vi "TestExample.vi"() -> ()   [LabVIEW 2012, in "Surelite I.lvlib"]
doc: "This is the instrument driver for the <INSTRUMENT NAME>. The VI Tree displays all the user-callable VIs of the instrument driver in an organized table."
uses:
  Surelite I.lvlib
panel:
  in  "ClearErr":bool
  out "error out":errorcluster
  out "Error Message":string[](array[string])
  in  "Check Error":bool
  in  "Shutdown":bool
  in  "Reset":bool
  in  "VISA resource name":refnum<visa-resource-name>="COM8"
  in  "Delay (us)":i32=200
  in  "RepRate (Hz)":sgl=10.0 min=0.1 max=30 step=0.1
  in  "Division":i32=1 min=1
  in  "Start? (F)":bool
  in  "Shutter (F)":bool
  in  "Voltage (kV)":sgl=1.08 min=0.9 max=1.2 step=0.01
  in  "Serial Configuration":T1={"Baud Rate"=9600, "Parity"=0, "Data Bits"=8, "Stop Bits"=10, "Flow Control"=0} {"Flow Control" items=["None", "XON/XOFF", "RTS/CTS", "XON/XOFF & RTS/CTS", "DTR/DSR", "XON/XOFF & DTR/DSR"]; "Stop Bits" items=["1.0"=10, "1.5"=15, "2.0"=20]; "Data Bits" items=["7"=7, "8"=8]; "Parity" items=["None", "Odd", "Even", "Mark", "Space"]; "Baud Rate" items=["300"=300, "600"=600, "1200"=1200, "2400"=2400, "4800"=4800, "9600"=9600, "19200"=19200]}
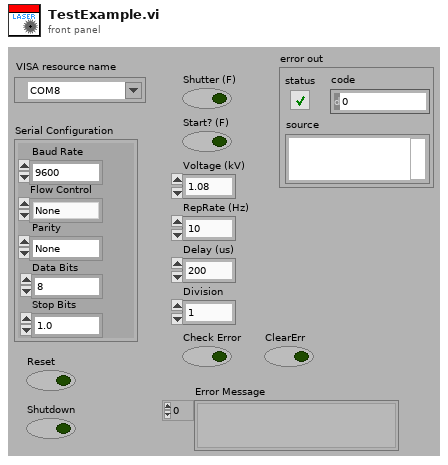
[diagram p1: front panel]
types:
  T1 = cluster{"Baud Rate":u32, "Parity":u16, "Data Bits":u16, "Stop Bits":u16, "Flow Control":u16}
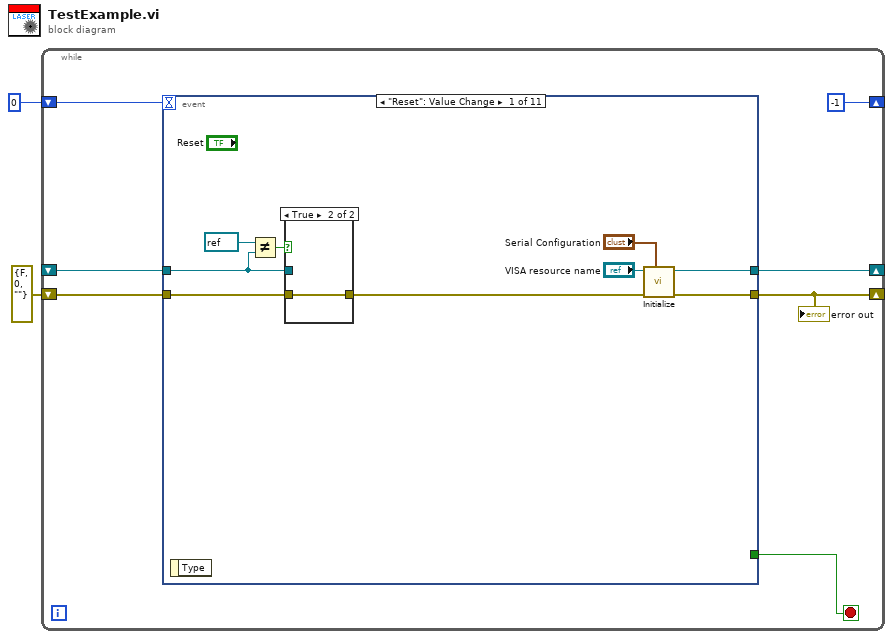
[diagram p0: block diagram]
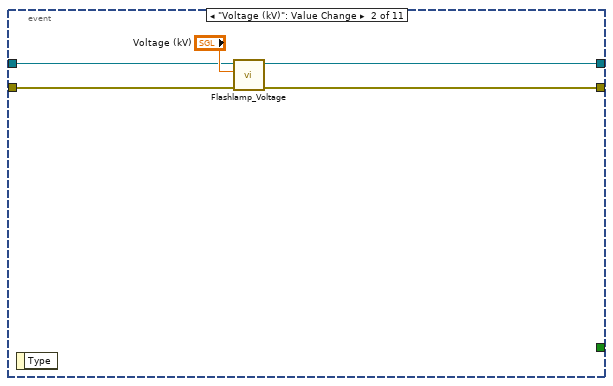
[diagram p3: hidden frame]
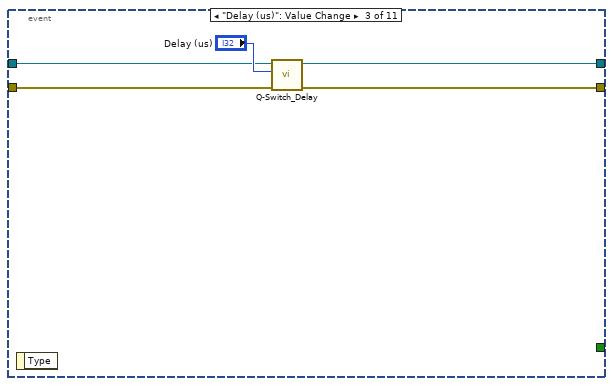
[diagram p4: hidden frame]
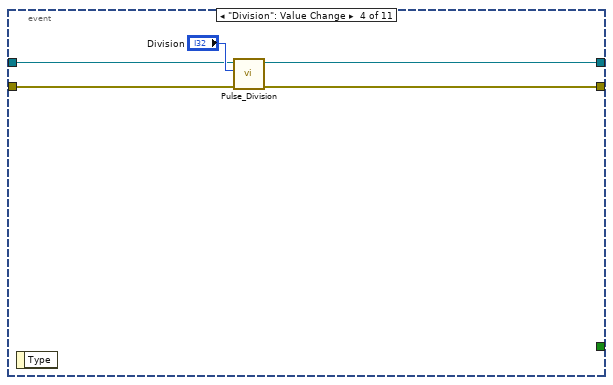
[diagram p5: hidden frame]
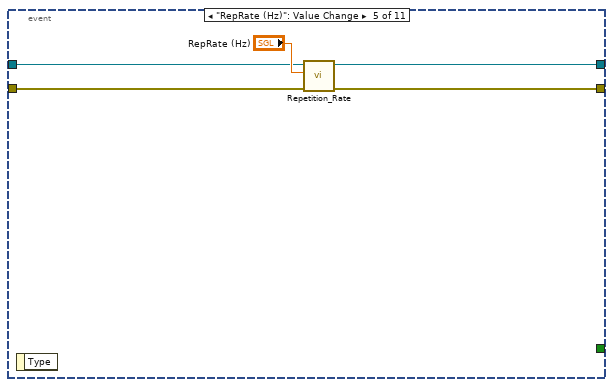
[diagram p6: hidden frame]
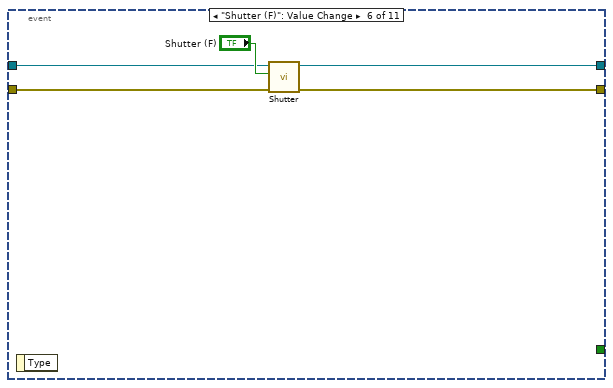
[diagram p7: hidden frame]
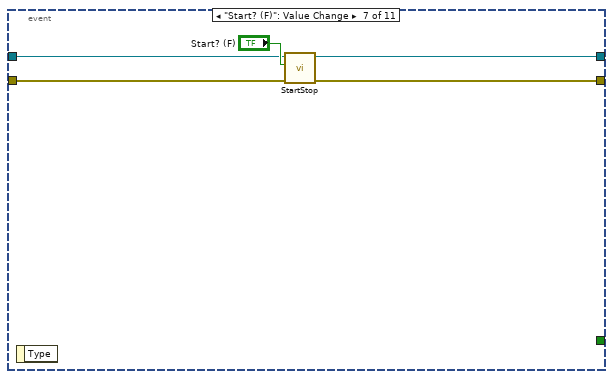
[diagram p8: hidden frame]
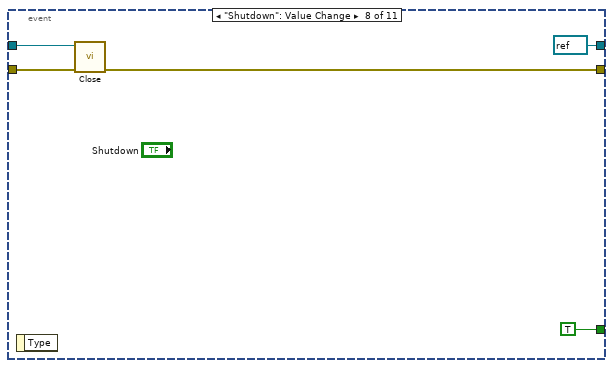
[diagram p9: hidden frame]
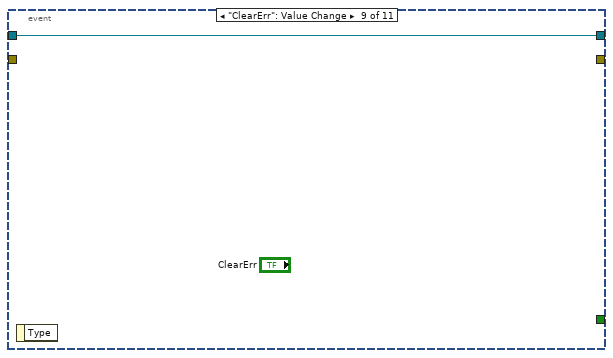
[diagram p10: hidden frame]
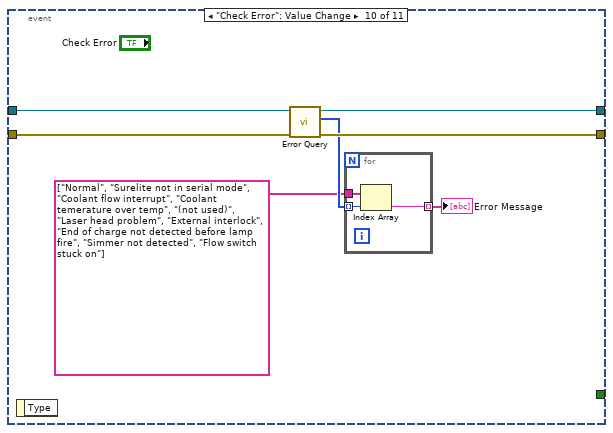
[diagram p11: hidden frame]
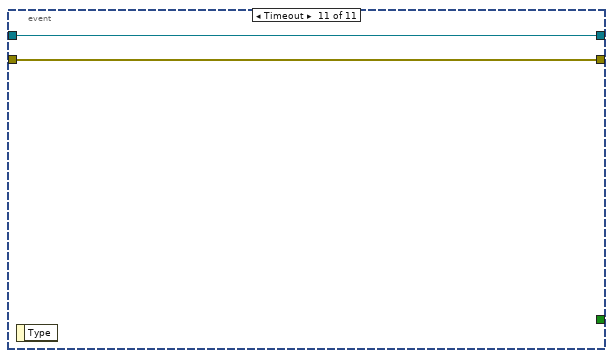
[diagram p12: hidden frame]
diagram:
  n1 = while {
    shift-right: [-1] -> _
    shift-left: 0 -> [w9]
    shift-right: [w7] -> _
    shift-left: _ -> [w6]
    shift-right: [w5] -> _
    shift-left: errorcluster {"status"=FALSE, "code"=0, "source"=""} ("error out") -> [w4]
    stop <- w3 stop-if-true
    n2 = event shown="[0] \"Reset\": Value Change" {
      selector: _ -> [_ _ _ _ _ _ _ _ _ _ _]
      dyn-events: _ -> [_ _ _ _ _ _ _ _ _ _ _]
      timeout: w9 -> [_ _ _ _ _ _ _ _ _ _ _]
      tunnel: [w16 w23 w28 w33 w38 w43 w48 refnum<visa-resource-name> refnum ("VISA resource name out") w56 w60 w67] -> w7
      tunnel: w6 -> [w11 w24 w29 w34 w39 w44 w49 w52 w56 w62 w67]
      tunnel: [w14 w21 w26 w31 w36 w41 w46 w53 _ w61 w68] -> w5
      tunnel: w4 -> [w13 w22 w27 w32 w37 w42 w47 w54 _ w63 w68]
      tunnel: [_ _ _ _ _ _ _ TRUE _ _ _] -> w3
      event "Reset": Value Change {
        n3 = event-data() -> ()  [unwired: 1 in, 1 out]
        n4 = Not Equal?(x=refnum<visa-resource-name> refnum, y=w11) -> (x != y?=w12:bool)
        n5 = case shown="True" w12 {
          tunnel: w11 -> [_ _]
          tunnel: [w19 w20] -> w15
          tunnel: w13 -> [w19 w20]
          frame False {
          }
          frame True {
          }
        }
        n6 = call "Initialize.vi"("Serial Configuration"="Serial Configuration", "error in (no error)"=w15, "VISA resource name"="VISA resource name") -> ("error out"=w14:errorcluster, "VISA resource name out"=w16:refnum<visa-resource-name>)  [unwired: 7 in]
      }
      event "Voltage (kV)": Value Change {
        n7 = event-data() -> ()  [unwired: 1 in, 1 out]
        n8 = call "Flashlamp_Voltage.vi"("error in (no error)"=w22, "Voltage (kV)"="Voltage (kV)", "VISA resource name"=w24) -> ("error out"=w21:errorcluster, "VISA resource name out"=w23:refnum<visa-resource-name>)  [unwired: 7 in]
      }
      event "Delay (us)": Value Change {
        n9 = event-data() -> ()  [unwired: 1 in, 1 out]
        n10 = call "Q-Switch_Delay.vi"("error in (no error)"=w27, "Delay (us)"="Delay (us)", "VISA resource name"=w29) -> ("error out"=w26:errorcluster, "VISA resource name out"=w28:refnum<visa-resource-name>)  [unwired: 7 in]
      }
      event "Division": Value Change {
        n11 = event-data() -> ()  [unwired: 1 in, 1 out]
        n12 = call "Pulse_Division.vi"("error in (no error)"=w32, "Division"="Division", "VISA resource name"=w34) -> ("error out"=w31:errorcluster, "VISA resource name out"=w33:refnum<visa-resource-name>)  [unwired: 7 in]
      }
      event "RepRate (Hz)": Value Change {
        n13 = event-data() -> ()  [unwired: 1 in, 1 out]
        n14 = call "Repetition_Rate.vi"("error in (no error)"=w37, "RepRate (Hz)"="RepRate (Hz)", "VISA resource name"=w39) -> ("error out"=w36:errorcluster, "VISA resource name out"=w38:refnum<visa-resource-name>)  [unwired: 7 in]
      }
      event "Shutter (F)": Value Change {
        n15 = event-data() -> ()  [unwired: 1 in, 1 out]
        n16 = call "Shutter.vi"("error in (no error)"=w42, "Open? (F)"="Shutter (F)", "VISA resource name"=w44) -> ("error out"=w41:errorcluster, "VISA resource name out"=w43:refnum<visa-resource-name>)  [unwired: 7 in]
      }
      event "Start? (F)": Value Change {
        n17 = event-data() -> ()  [unwired: 1 in, 1 out]
        n18 = call "StartStop.vi"("error in (no error)"=w47, "Start? (F)"="Start? (F)", "VISA resource name"=w49) -> ("error out"=w46:errorcluster, "VISA resource name out"=w48:refnum<visa-resource-name>)  [unwired: 7 in]
      }
      event "Shutdown": Value Change {
        n19 = event-data() -> ()  [unwired: 1 in, 1 out]
        n20 = call "Close.vi"("error in (no error)"=w54, "VISA resource name"=w52) -> ("error out"=w53:errorcluster)  [unwired: 9 in]
      }
      event "ClearErr": Value Change {
        n21 = event-data() -> ()  [unwired: 1 in, 1 out]
      }
      event "Check Error": Value Change {
        n22 = event-data() -> ()  [unwired: 1 in, 1 out]
        n23 = call "Error Query.vi"("error in (no error)"=w63, "VISA resource name"=w62) -> ("error out"=w61:errorcluster, "Error Code"=w59:i32[], "VISA resource name out"=w60:refnum<visa-resource-name>)  [unwired: 6 in, 1 out]
        n24 = for {
          tunnel: w59 -> [w66] mode=indexing
          tunnel: string[] ["Normal", "Surelite not in serial mode", "Coolant flow interrupt", "Coolant temerature over temp", "(not used)", "Laser head problem", "External interlock", "End of charge not detected before lamp fire", "Simmer not detected", "Flow switch stuck on"] -> [w65]
          tunnel: [w64] -> w57 mode=indexing
          n25 = Index Array(array=w65, index=w66) -> (element=w64:string)
        }
        "Error Message" <- w57
      }
      event Timeout {
        n26 = event-data() -> ()  [unwired: 1 in, 1 out]
      }
    }
    "error out" <- w5
  }
